vi "Data handler-Live imaging protocol.vi"(0 "Image array":T7, 1 "Logging queue":refnum<queue>, 5 "Logging queue element in":T3={"Imaging Protocol"=enum."Live Imaging", "Number of Trials"=0, "Frame Size"=512, "# Averaged frames"=0, "Dwell time (us)"=0.0, "Index of Z-plane"=0, "Timelapse?"=FALSE, "Logging process is active"=FALSE, "Speed logging enabled"=FALSE, "tdms file ref"=refnum, "path"=path "", "Trial Number"=0, "Expected # points acquired"=FALSE, "Manually stopped"=FALSE, "Last trial"=FALSE, "Ch0 data"=[], "Ch1 data"=[], "Ref Data"=[], "Ref Frame Time"=[], "Image Time"=[], "Continuous Time"=[], "Ref X Length"=0, "Ref Y Length"=0, "# Ref Averaged frames"=0, "Ref Dwell time (us)"=0.0, "Points acquired"={"Ch0 last trial"=0, "Ch1 last trial"=0, "All trials"=0}, "HW Timings File"=refnum} {"Ref Dwell time (us)" format="%#.6g"; "Frame Size" items=["100X100"=100, "128X128"=128, "200X200"=200, "256X256"=256, "512X512"=512, "1024x1024"=1024, "2048x2048"=2048]; "Dwell time (us)" format="%#.6g"}, 9 "Live graph data queue in":T2, 11 "error in (no error)":errorcluster, 12 "Single Frame Data":T1, 13 "Frame completed/generate image":bool, 14 "RefFrame completed/generate image":bool) -> (15 "error out":errorcluster)   [LabVIEW 2020]
uses:
  User Interface/Queue/Live graphs queue/Typedefs/Live imaging queue element.ctl
  <vilib>/vision/Image Controls.llb/IMAQ Image.ctl
  Typedefs/Logging queue element.ctl
  Typedefs/Imaging Protocols enum.ctl
  Typedefs/Frame Size.ctl
  Typedefs/Acquired points count.ctl
  User Interface/Typedefs/Live graph data queue ref.ctl
  Typedefs/Frame data dual cluster.ctl
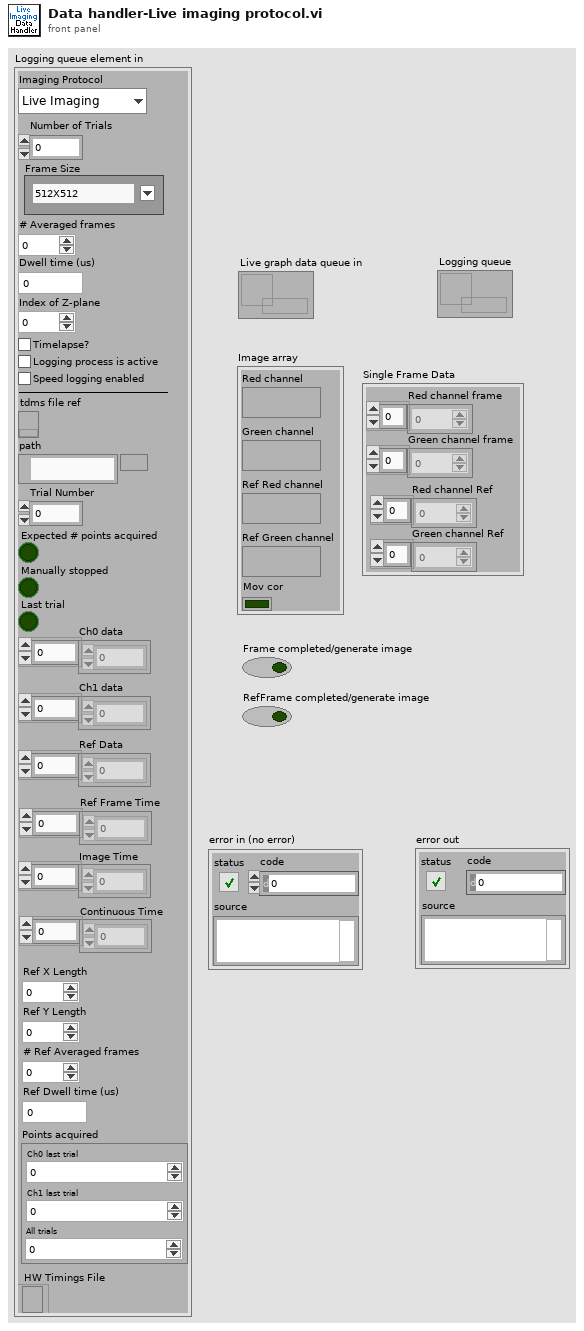
[diagram p1: front panel]
types:
  T1 = typedef "Frame data dual cluster.ctl" = cluster{"Red channel frame":dbl[], "Green channel frame":dbl[], "Red channel Ref":dbl[], "Green channel Ref":dbl[]}
  T2 = typedef "Live graph data queue ref.ctl" = refnum<queue>
  T3 = typedef "Logging queue element.ctl" = cluster{"Imaging Protocol":T4, "Number of Trials":u16, "Frame Size":T5, "# Averaged frames":u16, "Dwell time (us)":dbl, "Index of Z-plane":i32, "Timelapse?":bool, "Logging process is active":bool, "Speed logging enabled":bool, "tdms file ref":refnum<k34>, "path":path, "Trial Number":i32, "Expected # points acquired":bool, "Manually stopped":bool, "Last trial":bool, "Ch0 data":u32[], "Ch1 data":u32[], "Ref Data":u32[], "Ref Frame Time":u64[], "Image Time":u64[], "Continuous Time":u64[], "Ref X Length":u16, "Ref Y Length":u16, "# Ref Averaged frames":u16, "Ref Dwell time (us)":dbl, "Points acquired":T6, "HW Timings File":refnum<file>}
  T4 = typedef "Imaging Protocols enum.ctl" = enum16{"AOL Z-Stack", "Motor Z Stack", "Functional Acquisition", "Single Plane Acquisition", "Volume Acquisition", "Live Imaging", "Live Plane Imaging", "Live Volume Imaging"}
  T5 = typedef "Frame Size.ctl" = u16
  T6 = typedef "Acquired points count.ctl" = cluster{"Ch0 last trial":u64, "Ch1 last trial":u64, "All trials":u64}
  T7 = typedef "Live imaging queue element.ctl" = cluster{"Red channel":T8, "Green channel":T8, "Ref Red channel":T8, "Ref Green channel":T8, "Mov cor":bool}
  T8 = typedef "IMAQ Image.ctl" = refnum<image>
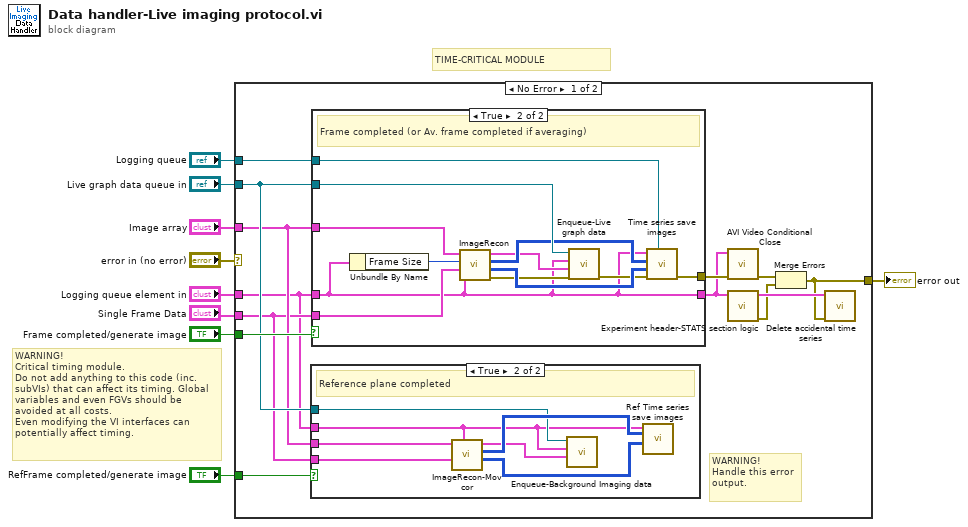
[diagram p0: block diagram]
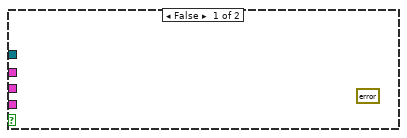
[diagram p2: hidden frame]
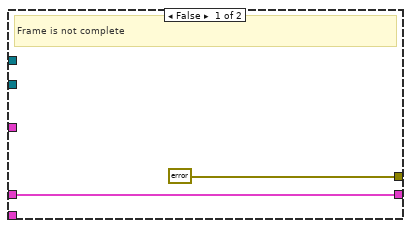
[diagram p3: hidden frame]
diagram:
  # "TIME-CRITICAL MODULE"
  # "WARNING!\nCritical timing module.\nDo not add anything to this code (inc. subVIs) that can affect its timing. Global variables and even FGVs should be avoided at all costs.\nEven modifying the VI interfaces can potentially affect timing."
  n1 = case shown="No Error" "error in (no error)" {
    selector: "error in (no error)" -> [_ w43]
    tunnel: [w10 w43] -> w9
    tunnel: "Image array" -> [w17 _]
    tunnel: "Logging queue element in" -> [w14 _]
    tunnel: "Live graph data queue in" -> [w18 _]
    tunnel: "Frame completed/generate image" -> [w21 _]
    tunnel: "Single Frame Data" -> [w16 _]
    tunnel: "Logging queue" -> [w20 _]
    tunnel: "RefFrame completed/generate image" -> [w19 _]
    frame No Error {
      # "WARNING!\nHandle this error\noutput."
      n2 = case shown="True" w19 {
        tunnel: w14 -> [_ w23]
        tunnel: w18 -> [_ w24]
        tunnel: w17 -> [_ w28]
        tunnel: w16 -> [_ w27]
        frame False {
          (unwired) errorcluster {"status"=FALSE, "code"=0, "source"=""} ("error out")
        }
        frame True {
          # "Reference plane completed"
          n3 = call "ImageRecon-Mov cor.vi"("Logging queue element in"=w23, "Data"=w27, "Image Array (in)"=w28) -> ("Ch1-Green-REF"=w25:i16[][], "Ch0-Red-REF"=w26:i16[][], "Image Array(out)"=w22:T7)  [unwired: 5 in, 1 out]
          n4 = call "Enqueue-Background Imaging data.vi"("Element to queue"=w22, "Logging queue element"=w23, "Live graph data queue in"=w24) -> ()  [unwired: 7 in, 2 out]
          n5 = call "Ref Time series save images.vi"("Ch1-Green-REF"=w25, "Ch0-Red-REF"=w26, "Logging queue element"=w23) -> ()  [unwired: 8 in, 1 out]
        }
      }
      n6 = case shown="True" w21 {
        tunnel: w17 -> [_ w42]
        tunnel: [errorcluster {"status"=FALSE, "code"=0, "source"=""} ("error out") w34] -> w15
        tunnel: w14 -> [w29 w31]
        tunnel: w16 -> [_ w41]
        tunnel: w18 -> [_ w40]
        tunnel: w20 -> [_ w32]
        tunnel: [w29 w31] -> w13
        frame False {
          # "Frame is not complete"
        }
        frame True {
          # "Frame completed (or Av. frame completed if averaging)"
          n7 = Unbundle By Name(w31) -> ("Frame Size"=w39:T5)
          n8 = call "ImageRecon.vi"("Logging queue element in"=w31, "Data"=w41, "Frame Size"=w39, "Image Array (in)"=w42) -> ("Error Out"=w36:errorcluster, "Ch1-Green"=w37:i16[][], "Ch0-Red"=w38:i16[][], "Image Array(out)"=w33:T7)  [unwired: 4 in]
          n9 = call "Enqueue-Live graph data.vi"("error in (no error)"=w36, "Element to queue"=w33, "Logging queue element"=w31, "Live graph data queue in"=w40) -> ("error out"=w35:errorcluster)  [unwired: 6 in, 1 out]
          n10 = call "Time series save images.vi"("Logging queue"=w32, "error in (no error)"=w35, "Ch1-Green"=w37, "Ch0-Red"=w38, "Logging queue element"=w31) -> ("error"=w34:errorcluster)  [unwired: 6 in]
        }
      }
      n11 = call "AVI Video Conditional Close.vi"("error in (no error)"=w15, "Logging queue element in"=w13) -> ("error out"=w12:errorcluster)  [unwired: 9 in]
      n12 = call "Experiment header-STATS section logic.vi"("Logging queue element"=w13) -> ("error out"=w11:errorcluster)  [unwired: 10 in]
      n13 = Merge Errors(w12, w11) -> (w10:errorcluster)
      n14 = call "Delete accidental time series.vi"("error in (no error)"=w10, "Logging queue element in"=w13) -> ()  [unwired: 10 in]
    }
    frame Error {
    }
  }
  "error out" <- w9
